vi "create_target_2.vi"(11 "Inputs":dbl[](array[numeric])) -> (3 "Target Array":dbl[](array[numeric]))   [LabVIEW 2015]
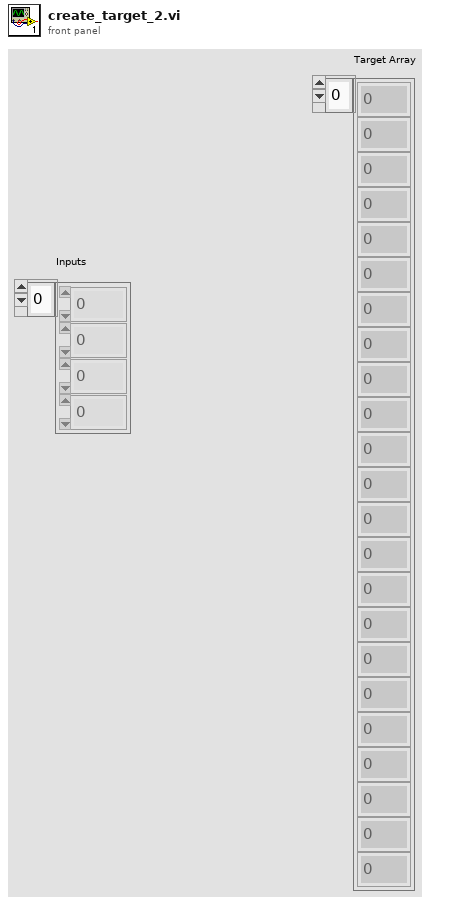
[diagram p1: front panel]
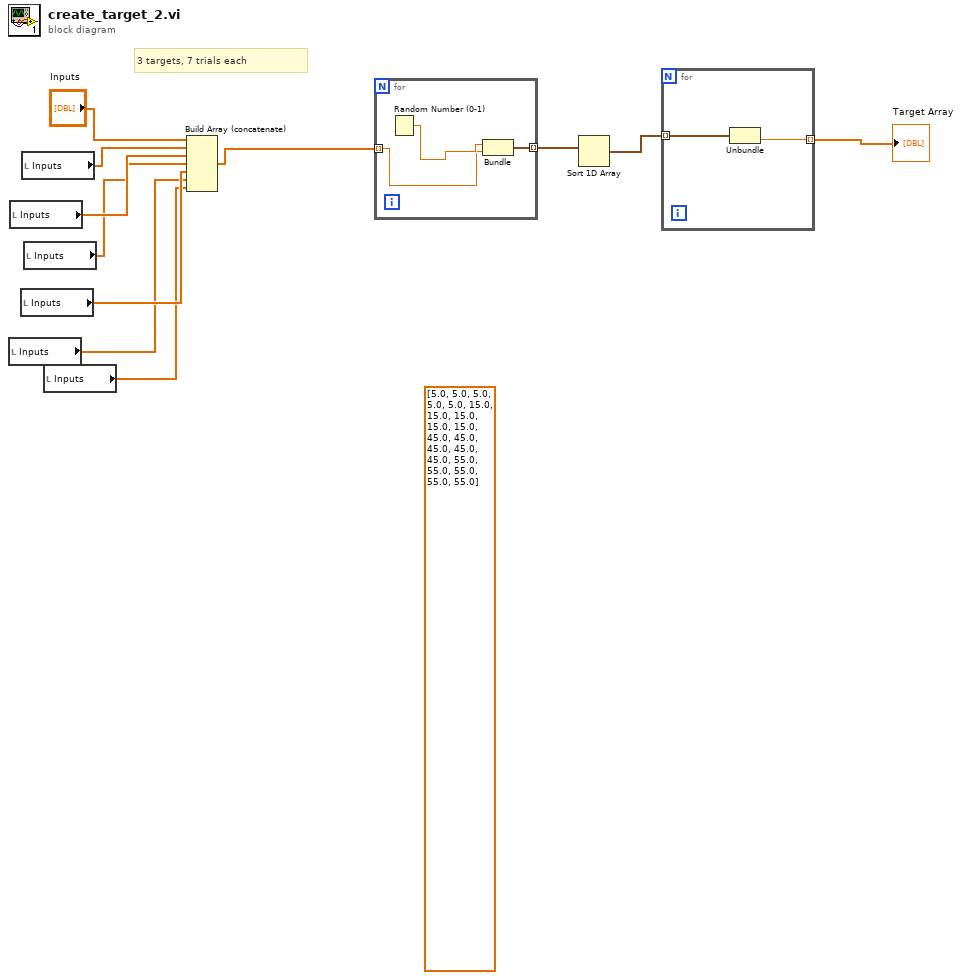
[diagram p0: block diagram]
diagram:
  (unwired) dbl[] [5.0, 5.0, 5.0, 5.0, 5.0, 15.0, 15.0, 15.0, 15.0, 15.0, 45.0, 45.0, 45.0, 45.0, 45.0, 55.0, 55.0, 55.0, 55.0, 55.0]
  # "3 targets, 7 trials each"
  n1 = local read "Inputs"() -> (w2:dbl[])
  n2 = local read "Inputs"() -> (w6:dbl[])
  n3 = local read "Inputs"() -> (w4:dbl[])
  n4 = local read "Inputs"() -> (w7:dbl[])
  n5 = local read "Inputs"() -> (w5:dbl[])
  n6 = local read "Inputs"() -> (w1:dbl[])
  n7 = Build Array (concatenate)("Inputs", w7, w6, w5, w4, w2, w1) -> (w3:dbl[])
  n8 = for {
    tunnel: w3 -> [w13] mode=indexing
    tunnel: [w12] -> w10 mode=indexing
    n9 = Random Number (0-1)() -> (number: 0 to 1=w14:dbl)
    n10 = Bundle("number: 0 to 1"=w14, "Numeric"=w13) -> (w12:cluster{"number: 0 to 1":dbl, "Numeric":dbl})  [unwired: 1 in]
  }
  n11 = Sort 1D Array(array=w10) -> (sorted array=w11:cluster{"number: 0 to 1":dbl, "Numeric":dbl}[])
  n12 = for {
    tunnel: w11 -> [w16] mode=indexing
    tunnel: [w15] -> w9 mode=indexing
    n13 = Unbundle(w16) -> ("Numeric"=w15:dbl)  [unwired: 1 out]
  }
  "Target Array" <- w9
